vi "Limit Yaw Angle.vi"(10 "u":dbl) -> (2 "output":dbl)   [LabVIEW 2016]
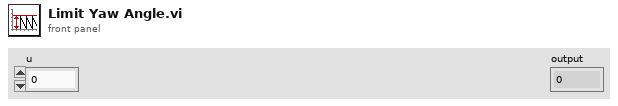
[diagram p1: front panel]
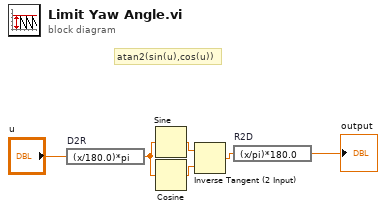
[diagram p0: block diagram]
diagram:
  # "atan2(sin(u),cos(u))"
  n1 = expression code="(x/180.0)*pi" "D2R"("u") -> (w6:dbl)
  n2 = Sine(x=w6) -> (sin(x)=w4:dbl)
  n3 = Cosine(x=w6) -> (cos(x)=w5:dbl)
  n4 = Inverse Tangent (2 Input)(1:w5, 2:w4) -> (0:w3:dbl)
  n5 = expression code="(x/pi)*180.0" "R2D"(w3) -> (→"output":dbl)
